vi "Variant_EmptyCluster.vi"(11 "Cluster Name":string) -> (3 "Empty Cluster":variant)   [LabVIEW 2013, in "OpenVariant.lvlib"]
uses:
  OpenVariant.lvlib
  <vilib>/Utility/GetType.llb/Type Descriptor I16 Array.ctl
  <vilib>/Utility/GetType.llb/Type Descriptor I16.ctl
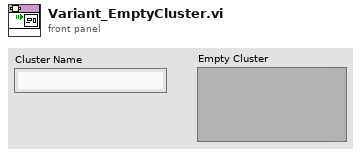
[diagram p1: front panel]
types:
  T1 = typedef "Type Descriptor I16 Array.ctl" = T2[]
  T2 = typedef "Type Descriptor I16.ctl" = i16
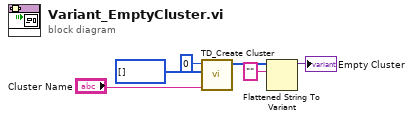
[diagram p0: block diagram]
diagram:
  n1 = call <vilib>:"TD_Create Cluster.vi"("Name"="Cluster Name", "Concatenated Elts"=T1 [], "N Elts"=i16 0) -> ("ClusterTD"=w5:T1)  [unwired: 8 in]
  n2 = Flattened String To Variant(6:"" ("data string"), 7:w5) -> (3:→"Empty Cluster":variant)  [unwired: 1 in, 1 out]
